vi "FGV_GEA2_Ref.vi"(0 "GEA2 Reference In":refnum<k24>, 7 "Action":enum16{"Set Ref", "Get Ref"}(ring), 11 "Error In":errorcluster) -> (4 "GEA2 Reference Out":refnum<k24>, 15 "Error Out":errorcluster)   [LabVIEW 2016]
doc: "This VI gets or sets the GEA2 reference."
uses:
  C:/Automation/DLLs/PC Dot Net/GeaCommunication.dll
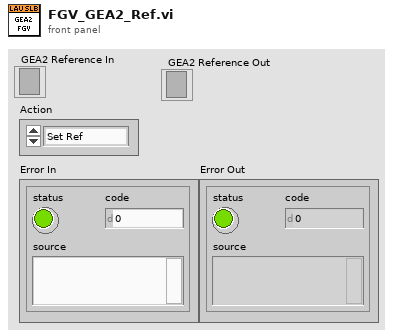
[diagram p1: front panel]
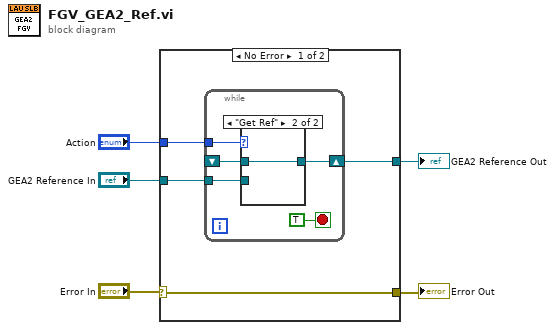
[diagram p0: block diagram]
diagram:
  n1 = case shown="No Error" "Error In" {
    selector: "Error In" -> [w6 w17]
    tunnel: "Action" -> [w9 _]
    tunnel: "GEA2 Reference In" -> [w8 _]
    tunnel: [w7 _] -> w3
    tunnel: [w6 w17] -> w1
    frame No Error {
      n2 = while {
        tunnel: w9 -> [w13]
        tunnel: w8 -> [w12]
        shift-right: [w11] -> w7
        shift-left: _ -> [w10]
        stop <- TRUE stop-if-true
        n3 = case shown="\"Get Ref\"" w13 {
          tunnel: w12 -> [w15 _]
          tunnel: [w15 w16] -> w11
          tunnel: w10 -> [_ w16]
          frame "Set Ref" {
          }
          frame "Get Ref" {
          }
        }
      }
    }
    frame Error {
    }
  }
  "GEA2 Reference Out" <- w3
  "Error Out" <- w1
